vi "Average_P_step_2.vi"(6 "Averaged P(B) in":dbl[][](array[numeric]), 7 "B array":dbl[](array[numeric]), 10 "Counter":i8, 11 "Stepped P(B)":dbl[][](array[numeric])) -> (3 "Averaged P(B) out":dbl[][](array[numeric]))   [LabVIEW 2015]
panel:
  out "element":dbl
  out "Offset array dn":dbl[](array[numeric])
  out "P(B) Stepped 2":cluster{"B array":dbl[], "Stepped P(B)":dbl[]}[](graph)
  out "P(B) Averaged":cluster{"B array":dbl[], dbl[]}[](graph)
  out "P(B) Offset removed":cluster{"B array":dbl[], "Stepped P(B)":dbl[]}[](graph)
  out "P(B) Stepped":cluster{"B array":dbl[], dbl[]}[](graph)
  out "OffsetRemoved":dbl[][](array[numeric])
  out "Offset array":dbl[](array[numeric])
  out "size(s)":i32
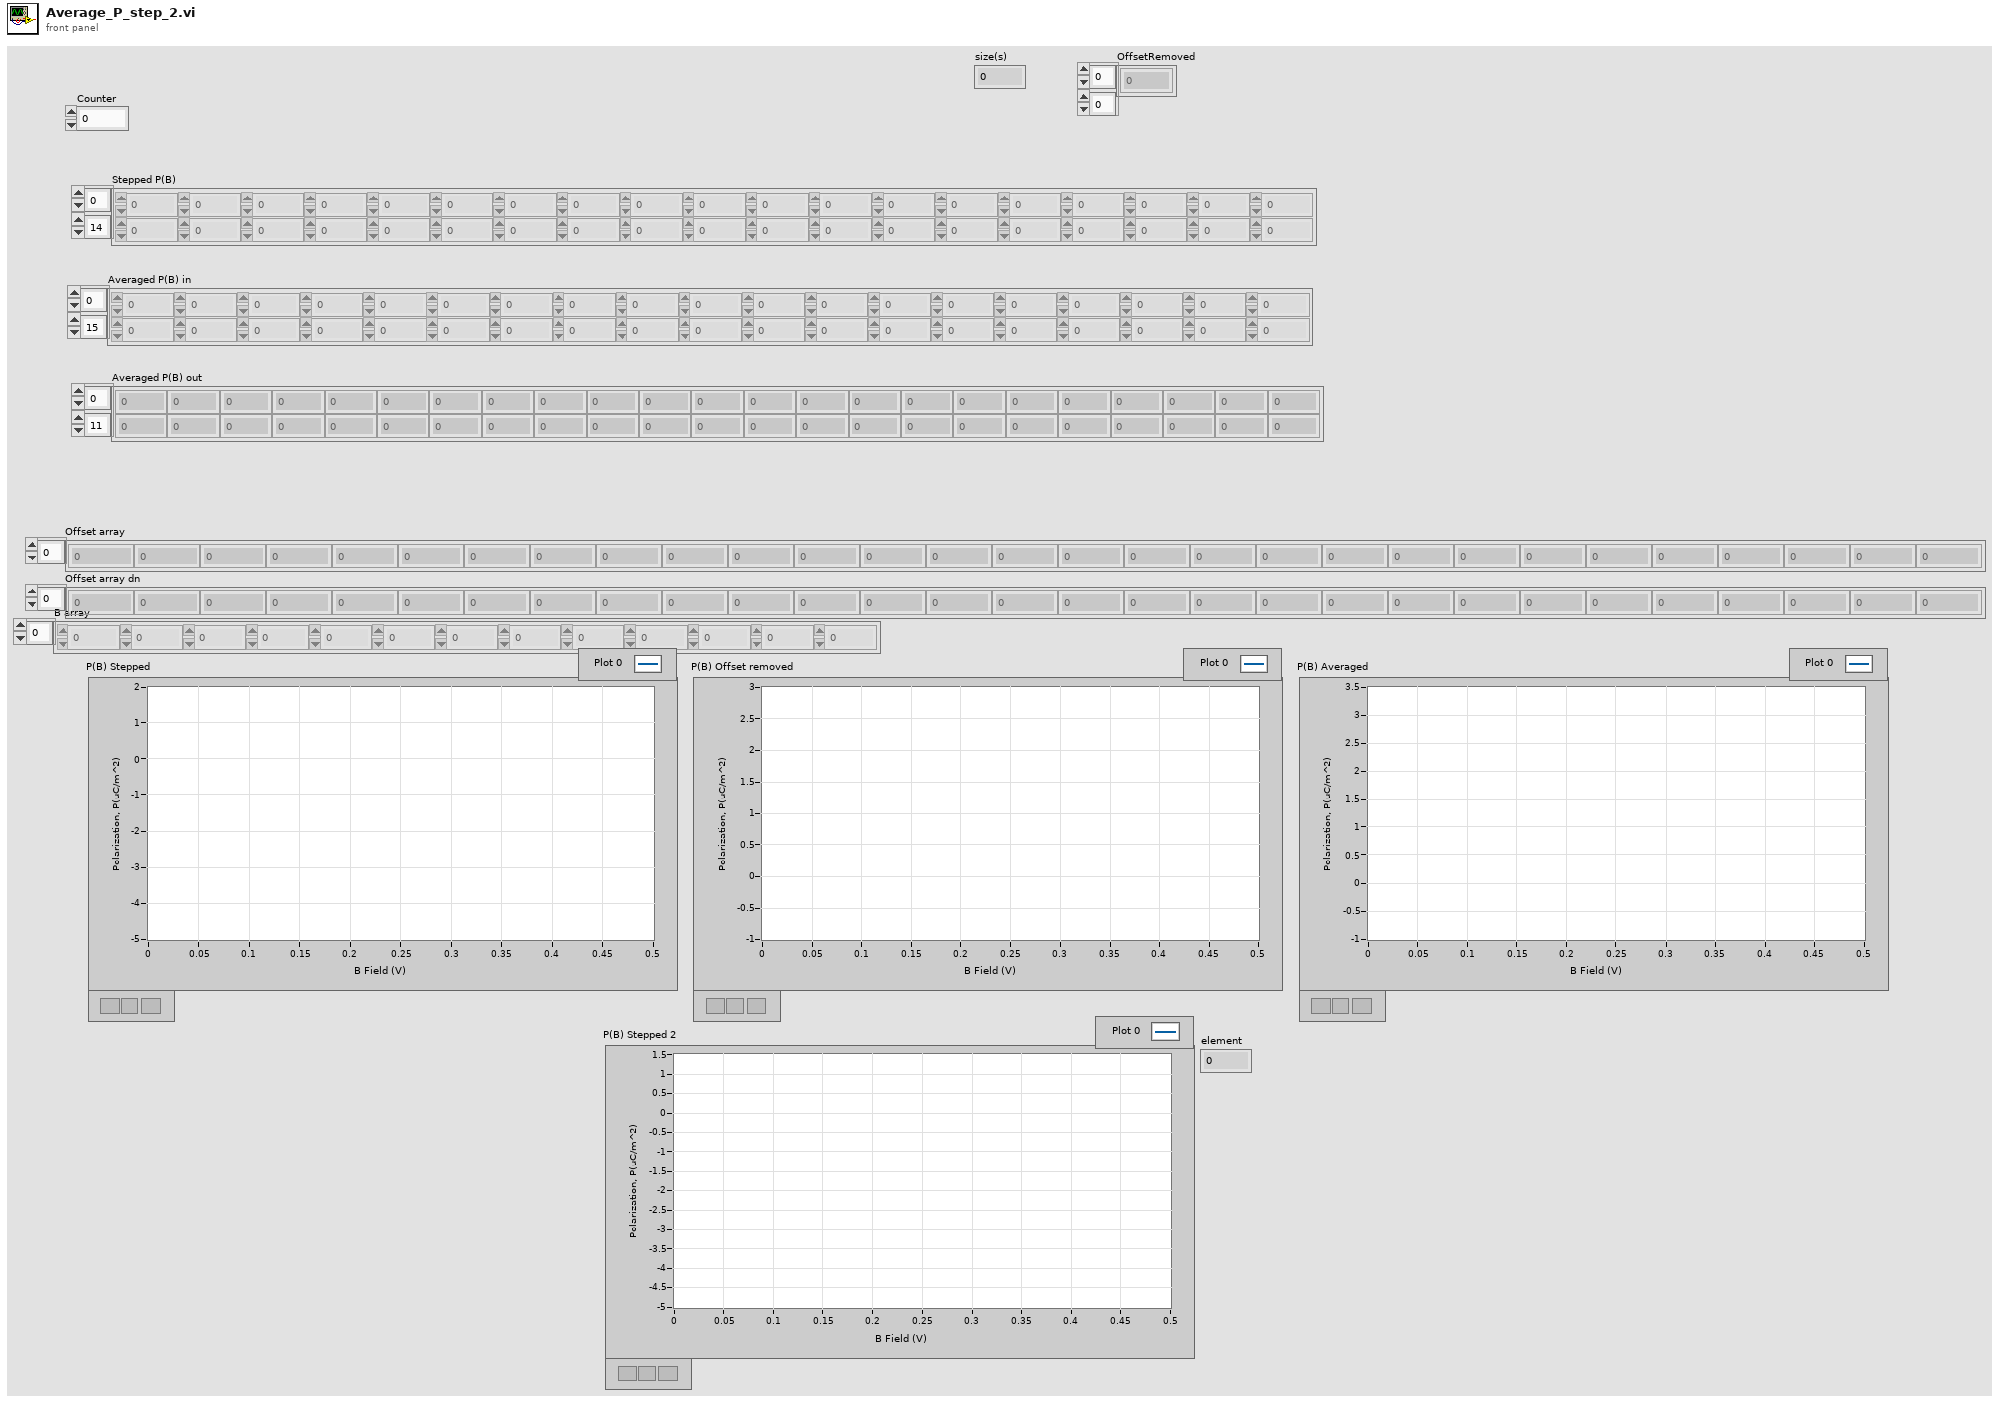
[diagram p1: front panel]
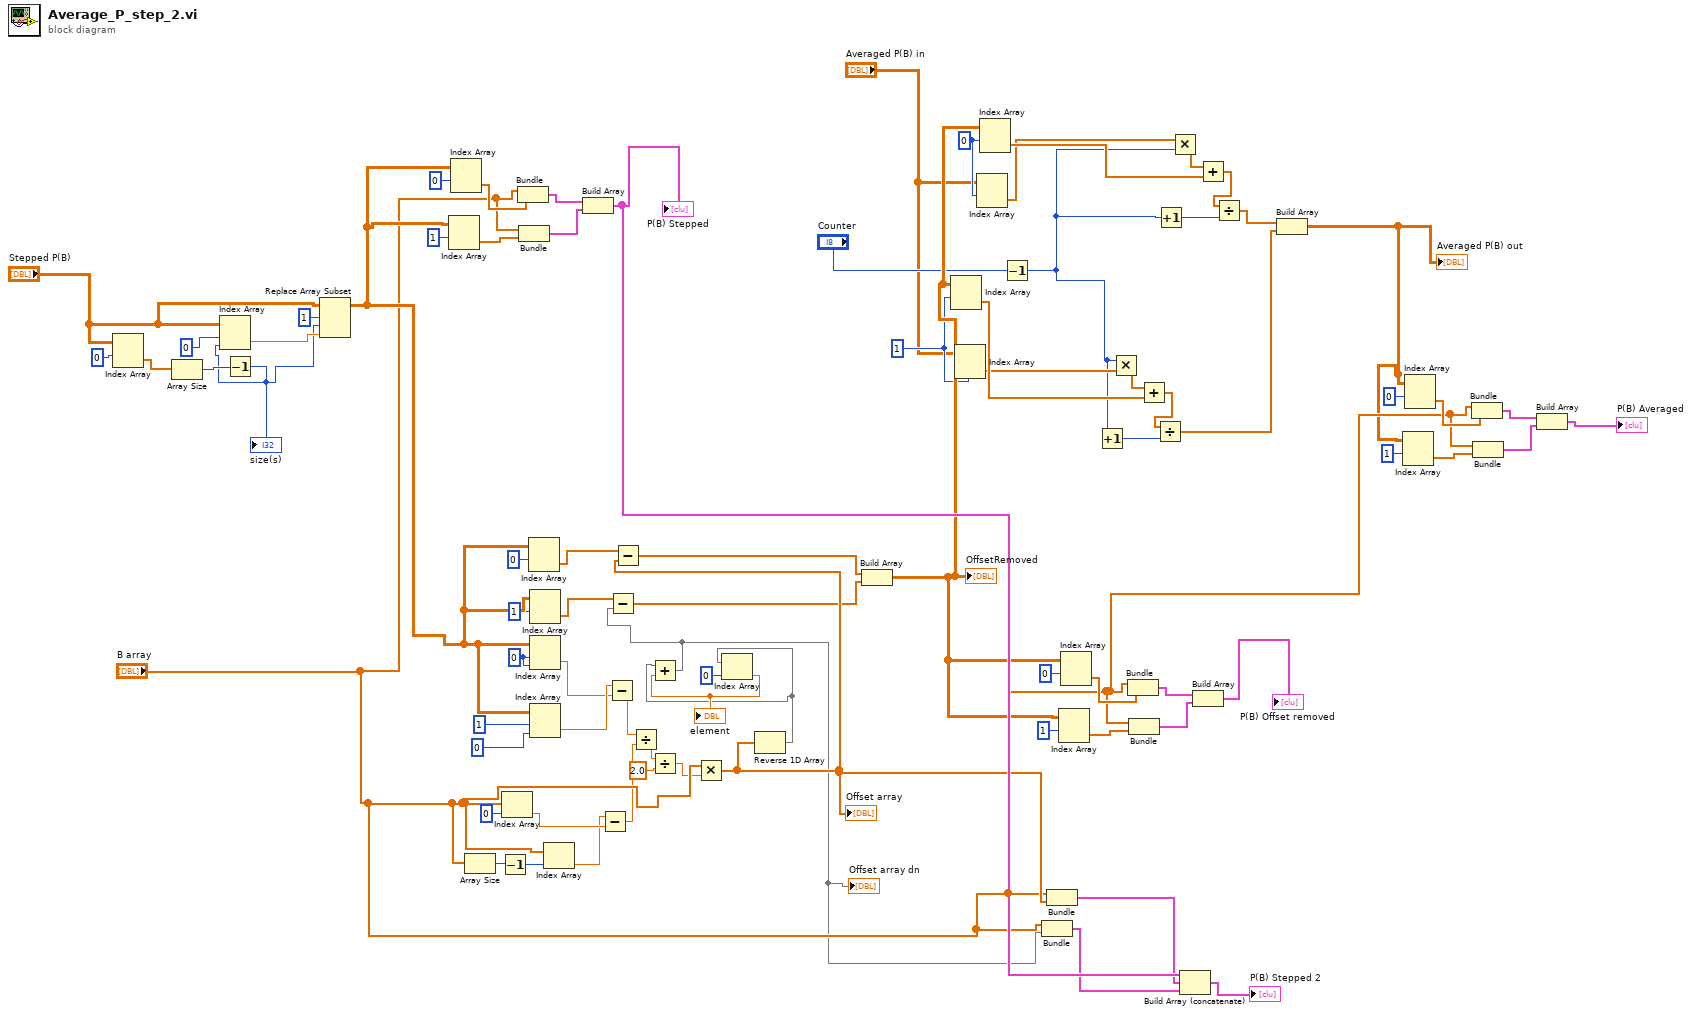
[diagram p0: block diagram]
diagram:
  w10 = 0 ("index (row)")
  w39 = 0 ("index (row)")
  w15 = 1 ("f")
  n1 = Index Array(array="Stepped P(B)", index (row)=0) -> (element=w74:dbl[])  [unwired: 1 in]
  n2 = Array Size(array=w74) -> (size(s)=w71:i32)
  n3 = Decrement(x=w71) -> (x-1=w69:i32)
  "size(s)" <- w69
  n4 = Index Array(array="Stepped P(B)", index (row)=0, index (col)=w69) -> (element=w72:dbl)
  n5 = Replace Array Subset(array="Stepped P(B)", new element=w72, index (row)=1, index (col)=w69) -> (w48:dbl[][])
  n6 = Index Array(array=w48, index (row)=1) -> (element=w64:dbl[])  [unwired: 1 in]
  n7 = Index Array(array=w48, index (row)=0) -> (element=w65:dbl[])  [unwired: 1 in]
  n8 = Array Size(array="B array") -> (size(s)=w25:i32)
  n9 = Decrement(x=w25) -> (x-1=w33:i32)
  n10 = Index Array(array="B array", index=0) -> (element=w32:dbl)
  n11 = Bundle("B array"="B array", "Stepped P(B)"=w65) -> (w63:cluster{"B array":dbl[], "Stepped P(B)":dbl[]})  [unwired: 1 in]
  n12 = Bundle("B array"="B array", "Stepped P(B)"=w64) -> (w62:cluster{"B array":dbl[], "Stepped P(B)":dbl[]})  [unwired: 1 in]
  n13 = Index Array(array=w48, index (row)=0) -> (element=w24:dbl[])  [unwired: 1 in]
  n14 = Index Array(array=w48, index (row)=1) -> (element=w23:dbl[])  [unwired: 1 in]
  n15 = Index Array(array=w48, index (row)=w39, index (col)=w39) -> (element=w35:dbl)
  n16 = Index Array(array=w48, index (row)=1, index (col)=0 ("index (row)")) -> (element=w36:dbl)
  n17 = Index Array(array="B array", index=w33) -> (element=w19:dbl)
  n18 = Build Array(w63, w62) -> (w47:cluster{"B array":dbl[], "Stepped P(B)":dbl[]}[])
  "P(B) Stepped" <- w47
  n19 = Subtract(x=w19, y=w32) -> (x-y=w28:dbl)
  n20 = Subtract(x=w36, y=w35) -> (x-y=w29:dbl)
  n21 = Divide(x=w29, y=w28) -> (x/y=w27:dbl)
  n22 = Divide(x=w27, y=2.0) -> (x/y=w20:dbl)
  n23 = Multiply(x="B array", y=w20) -> (x*y=w46:dbl[])
  "Offset array" <- w46
  n24 = Subtract(x=w24, y=w46) -> (x-y=w22:dbl[])
  n25 = Reverse 1D Array(array=w46) -> (reversed array=w16:dbl[])
  n26 = Index Array(array=w16, index=0) -> (element=w17:dbl)
  "element" <- w17
  n27 = Add(x=w16, y=w17) -> (x+y=w44:dbl[])
  "Offset array dn" <- w44
  n28 = Subtract(x=w23, y=w44) -> (x-y=w21:dbl[])
  n29 = Build Array(w22, w21) -> (w40:dbl[][])
  "OffsetRemoved" <- w40
  n30 = Index Array(array=w40, index (row)=w15) -> (element=w79:dbl[])  [unwired: 1 in]
  n31 = Index Array(array="Averaged P(B) in", index (row)=w15) -> (element=w4:dbl[])  [unwired: 1 in]
  n32 = Index Array(array="Averaged P(B) in", index (row)=w10) -> (element=w8:dbl[])  [unwired: 1 in]
  n33 = Index Array(array=w40, index (row)=w10) -> (element=w9:dbl[])  [unwired: 1 in]
  n34 = Decrement(x="Counter") -> (x-1=w1:i8)
  n35 = Bundle("B array"="B array", w44) -> (w42:cluster{"B array":dbl[], dbl[]})  [unwired: 1 in]
  n36 = Bundle("B array"="B array", w46) -> (w43:cluster{"B array":dbl[], dbl[]})  [unwired: 1 in]
  n37 = Index Array(array=w40, index (row)=1) -> (element=w58:dbl[])  [unwired: 1 in]
  n38 = Index Array(array=w40, index (row)=0) -> (element=w57:dbl[])  [unwired: 1 in]
  n39 = Increment(x=w1) -> (x+1=w77:i8)
  n40 = Multiply(x=w1, y=w4) -> (x*y=w76:dbl[])
  n41 = Bundle("B array"="B array", w57) -> (w59:cluster{"B array":dbl[], dbl[]})  [unwired: 1 in]
  n42 = Bundle("B array"="B array", w58) -> (w60:cluster{"B array":dbl[], dbl[]})  [unwired: 1 in]
  n43 = Add(x=w76, y=w79) -> (x+y=w78:dbl[])
  n44 = Divide(x=w78, y=w77) -> (x/y=w6:dbl[])
  n45 = Increment(x=w1) -> (x+1=w13:i8)
  n46 = Multiply(x=w8, y=w1) -> (x*y=w14:dbl[])
  n47 = Build Array (concatenate)(w47, w43, w42) -> (→"P(B) Stepped 2":cluster{"B array":dbl[], "Stepped P(B)":dbl[]}[])
  n48 = Build Array(w59, w60) -> (→"P(B) Offset removed":cluster{"B array":dbl[], dbl[]}[])
  n49 = Add(x=w14, y=w9) -> (x+y=w12:dbl[])
  n50 = Divide(x=w12, y=w13) -> (x/y=w7:dbl[])
  n51 = Build Array(w7, w6) -> (w3:dbl[][])
  "Averaged P(B) out" <- w3
  n52 = Index Array(array=w3, index (row)=1) -> (element=w51:dbl[])  [unwired: 1 in]
  n53 = Index Array(array=w3, index (row)=0) -> (element=w52:dbl[])  [unwired: 1 in]
  n54 = Bundle("B array"="B array", w52) -> (w50:cluster{"B array":dbl[], dbl[]})  [unwired: 1 in]
  n55 = Bundle("B array"="B array", w51) -> (w49:cluster{"B array":dbl[], dbl[]})  [unwired: 1 in]
  n56 = Build Array(w50, w49) -> (→"P(B) Averaged":cluster{"B array":dbl[], dbl[]}[])
